vi "main_ctrl.vi"() -> ()   [LabVIEW 2020]
doc: "Use this template to build a simple state machine design pattern. Each state executes code and determines which state to transition to."
uses:
  Type Defs/rs2_ctrl_panel.ctl
  <vilib>/Instr/_visa.llb/VISA Configure Serial Port (Instr).vi
panel:
  in  "Stop":bool
  out "Status":string
  in  "Device Control-In":T1={"Stimulation Parameters"={"Amplitude (mA)"={"A1"=1, "A2"=0, "A3"=0, "A4"=0, "A5"=0, "A6"=0, "A7"=0, "A8"=0}, "Pulse Width (µs)"={"PW1"=20, "PW2"=20, "PW3"=20, "PW4"=20, "PW5"=20, "PW6"=20, "PW7"=20, "PW8"=20}, "Stimulation Mode"={"M1"=0, "M2"=0, "M3"=0, "M4"=0, "M5"=0, "M6"=0, "M7"=0, "M8"=0}}, "Waveform Parameters"={"Low Frequency Factor"=0, "Main Stim Interval [ms]"=8.0, "Interpulse Interval [ms]"=0, "Channel Execution"=0}, "Active channels"={"C1"=FALSE, "C2"=FALSE, "C3"=FALSE, "C4"=FALSE, "C5"=FALSE, "C6"=FALSE, "C7"=FALSE, "C8"=FALSE}, "LF Active Channels"={"LF1"=FALSE, "LF2"=FALSE, "LF3"=FALSE, "LF4"=FALSE, "LF5"=FALSE, "LF6"=FALSE, "LF7"=FALSE, "LF8"=FALSE}, "Device Control"={"VISA resource name"=""}} {"Stimulation Parameters"."Amplitude (mA)"."A1" max=130; "Stimulation Parameters"."Amplitude (mA)"."A2" max=130; "Stimulation Parameters"."Amplitude (mA)"."A3" max=130; "Stimulation Parameters"."Amplitude (mA)"."A4" max=130; "Stimulation Parameters"."Amplitude (mA)"."A5" max=130; "Stimulation Parameters"."Amplitude (mA)"."A6" max=130; "Stimulation Parameters"."Amplitude (mA)"."A7" max=130; "Stimulation Parameters"."Amplitude (mA)"."A8" max=130; "Stimulation Parameters"."Pulse Width (µs)"."PW1" min=20 max=500; "Stimulation Parameters"."Pulse Width (µs)"."PW2" min=20 max=500; "Stimulation Parameters"."Pulse Width (µs)"."PW3" min=20 max=500; "Stimulation Parameters"."Pulse Width (µs)"."PW4" min=20 max=500; "Stimulation Parameters"."Pulse Width (µs)"."PW5" min=20 max=500; "Stimulation Parameters"."Pulse Width (µs)"."PW6" min=20 max=500; "Stimulation Parameters"."Pulse Width (µs)"."PW7" min=20 max=500; "Stimulation Parameters"."Pulse Width (µs)"."PW8" min=20 max=500; "Stimulation Parameters"."Stimulation Mode"."M8" items=["Singlet", "Doublet", "Triplet"]; "Stimulation Parameters"."Stimulation Mode"."M7" items=["Singlet", "Doublet", "Triplet"]; "Stimulation Parameters"."Stimulation Mode"."M6" items=["Singlet", "Doublet", "Triplet"]; "Stimulation Parameters"."Stimulation Mode"."M5" items=["Singlet", "Doublet", "Triplet"]; "Stimulation Parameters"."Stimulation Mode"."M4" items=["Singlet", "Doublet", "Triplet"]; "Stimulation Parameters"."Stimulation Mode"."M3" items=["Singlet", "Doublet", "Triplet"]; "Stimulation Parameters"."Stimulation Mode"."M2" items=["Singlet", "Doublet", "Triplet"]; "Stimulation Parameters"."Stimulation Mode"."M1" items=["Singlet", "Doublet", "Triplet"]; "Waveform Parameters"."Channel Execution" items=["Fixed Interval", "ASAP"]}
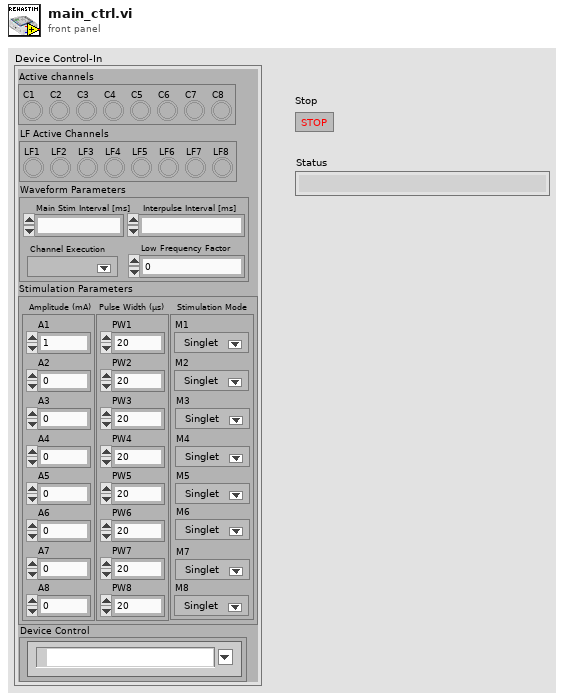
[diagram p1: front panel]
types:
  T1 = typedef "rs2_ctrl_panel.ctl" = cluster{"Stimulation Parameters":cluster{"Amplitude (mA)":cluster{"A1":u8, "A2":u8, "A3":u8, "A4":u8, "A5":u8, "A6":u8, "A7":u8, "A8":u8}, "Pulse Width (µs)":cluster{"PW1":u16, "PW2":u16, "PW3":u16, "PW4":u16, "PW5":u16, "PW6":u16, "PW7":u16, "PW8":u16}, "Stimulation Mode":cluster{"M1":u8, "M2":u8, "M3":u8, "M4":u8, "M5":u8, "M6":u8, "M7":u8, "M8":u8}}, "Waveform Parameters":cluster{"Low Frequency Factor":u8, "Main Stim Interval [ms]":fxp<+,32,11>, "Interpulse Interval [ms]":u8, "Channel Execution":u8}, "Active channels":cluster{"C1":bool, "C2":bool, "C3":bool, "C4":bool, "C5":bool, "C6":bool, "C7":bool, "C8":bool}, "LF Active Channels":cluster{"LF1":bool, "LF2":bool, "LF3":bool, "LF4":bool, "LF5":bool, "LF6":bool, "LF7":bool, "LF8":bool}, "Device Control":cluster{"VISA resource name":refnum<visa-resource-name>}}
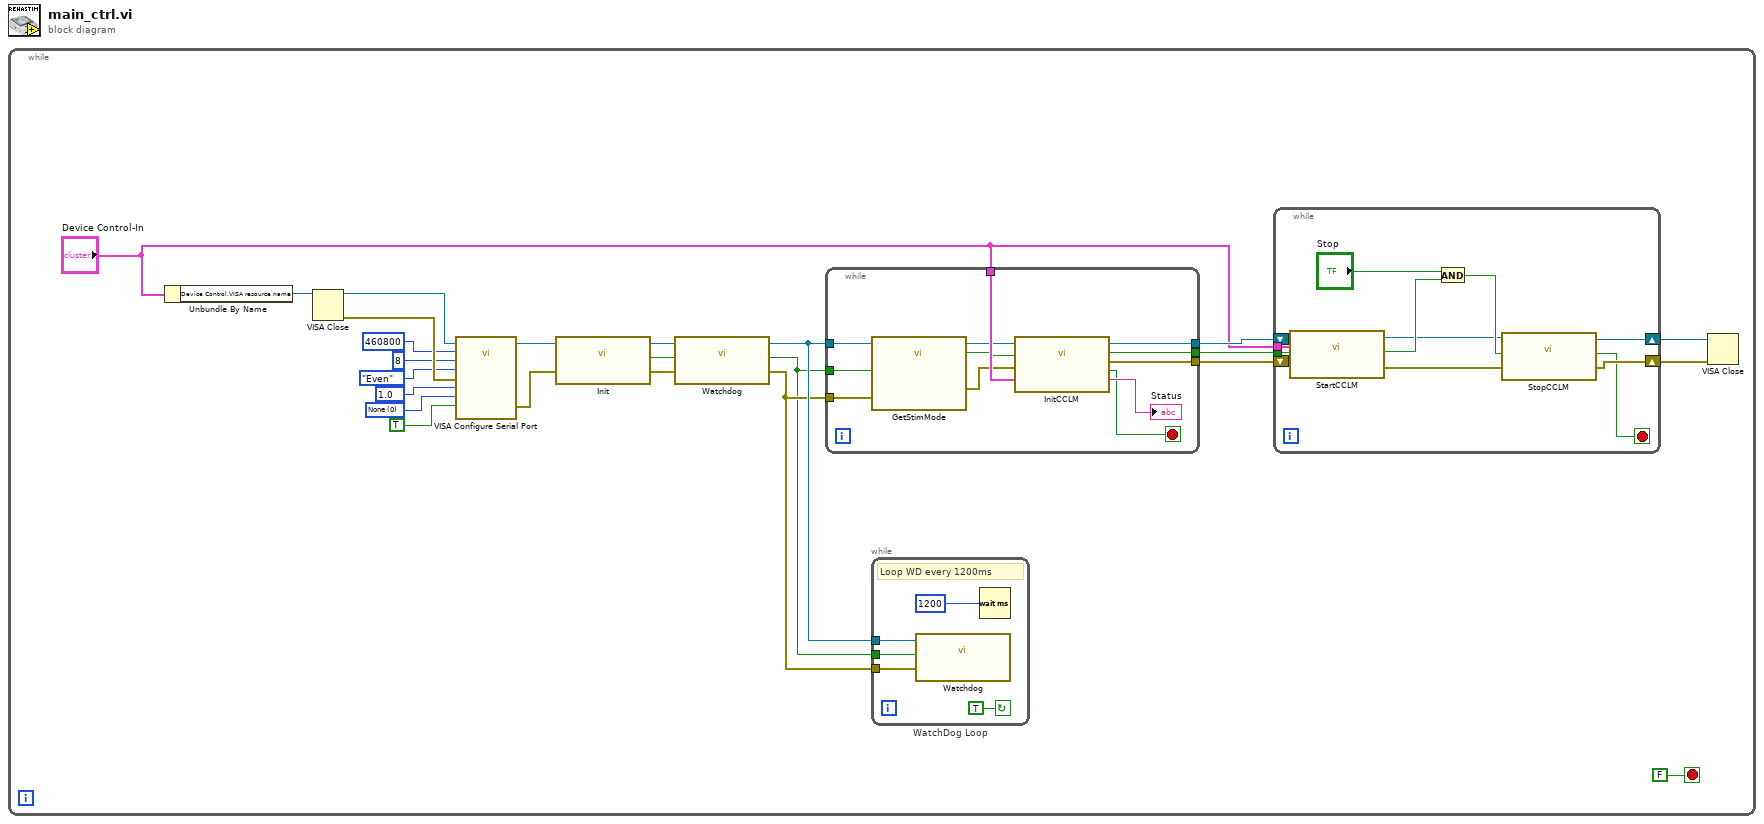
[diagram p0: block diagram]
diagram:
  n1 = while {
    stop <- FALSE stop-if-true
    w14 = u16 10 items=["1.0"=10, "1.5"=15, "2.0"=20] ("stop bits (10: 1 bit)")
    w15 = u16 0 items=["None", "XON/XOFF", "RTS/CTS", "XON/XOFF & RTS/CTS", "DTR/DSR", "XON/XOFF & DTR/DSR"] ("flow control (0:none)")
    n2 = Unbundle By Name("Device Control-In") -> ("Device Control.VISA resource name"=w20:refnum<visa-resource-name>)
    n3 = VISA Close(VISA resource name=w20) -> (error out=w23:errorcluster)  [unwired: 1 in]
    n4 = call-poly "VISA Configure Serial Port"("VISA resource name"=w20, "Enable Termination\nChar (T)"=TRUE ("Enable Termination\nChar (T)"), "baud rate (9600)"=u32 460800, "data bits (8)"=u16 8, "parity (0:none)"=enum16{"None", "Odd", "Even", "Mark", "Space"}."Even", "error in (no error)"=w23, "stop bits (10: 1 bit)"=w14, "flow control (0:none)"=w15) -> ("VISA resource name out"=w22:refnum<visa-resource-name>, "error out"=w21:errorcluster)  [unwired: 6 in]
    n5 = call "Init.vi"("VISA resource name"=w22, "error in (no error)"=w21) -> ("VISA resource name out"=w13:refnum<visa-resource-name>, "Init Status"=w11:bool, "error out"=w12:errorcluster)  [unwired: 11 in]
    n6 = call "Watchdog.vi"("COM Port Select"=w13, "Enable-In"=w11, "error in (no error)"=w12) -> ("VISA resource name out"=w10:refnum<visa-resource-name>, "WatchDog Status"=w8:bool, "error out"=w9:errorcluster)  [unwired: 10 in]
    n7 = while {
      tunnel: "Device Control-In" -> [w47]
      tunnel: w10 -> [w44]
      tunnel: w9 -> [w43]
      tunnel: w8 -> [w42]
      tunnel: [w38] -> w7
      tunnel: [w37] -> w6
      tunnel: [w36] -> w4
      stop <- w39 stop-if-true
      n8 = call "GetStimMode.vi"("VISA Resource Name"=w44, "DeviceInitializationEnable"=w42, "error in (no error)"=w43) -> ("VISA resource name out"=w46:refnum<visa-resource-name>, "Start Mode"=w41:bool, "error out"=w45:errorcluster)  [unwired: 6 in, 4 out]
      n9 = call "InitCCLM.vi"("COM Port Select"=w46, "StartModeEnable"=w41, "error in (no error)"=w45, "User control"=w47) -> ("Status"=→"Status":string, "VISA resource name out"=w38:refnum<visa-resource-name>, "Stimulation Initialized"=w37:bool, "CCLM Initialization Error"=w39:bool, "error out"=w36:errorcluster)  [unwired: 7 in]
    }
    n10 = while "WatchDog Loop" {
      tunnel: w10 -> [w50]
      tunnel: w9 -> [w49]
      tunnel: w8 -> [w48]
      stop <- TRUE continue-if-true
      # "Loop WD every 1200ms"
      n11 = call "Watchdog.vi"("COM Port Select"=w50, "Enable-In"=w48, "error in (no error)"=w49) -> ()  [unwired: 10 in, 3 out]
      n12 = Wait (ms)(milliseconds to wait=u32 1200) -> ()  [unwired: 1 out]
    }
    n13 = while {
      tunnel: w6 -> [w34]
      tunnel: "Device Control-In" -> [w33]
      shift-right: [w28] -> w3
      shift-left: w7 -> [w35]
      shift-right: [w27] -> w2
      shift-left: w4 -> [w32]
      stop <- w25 stop-if-true
      n14 = call "StartCCLM.vi"("VISA resource name"=w35, "Device Control-In 2"=w33, "StimInitializationEnable"=w34, "error in (no error)"=w32) -> ("VISA resource name out"=w29:refnum<visa-resource-name>, "Stimulation Started"=w30:bool, "error out"=w26:errorcluster)  [unwired: 9 in]
      n15 = And(x="Stop", y=w30) -> (x .and. y?=w31:bool)
      n16 = call "StopCCLM.vi"("VISA Resource Name"=w29, "Stop Stimulation"=w31, "error in (no error)"=w26) -> ("VISA resource name out"=w28:refnum<visa-resource-name>, "Stimulation Stopped"=w25:bool, "error out"=w27:errorcluster)  [unwired: 10 in]
    }
    n17 = VISA Close(VISA resource name=w3, error in (no error)=w2) -> ()  [unwired: 1 out]
  }
